vi "Invert_Binary.vi"(8 "error in (no error)":errorcluster, 11 "Input Result from Terminal":string) -> (0 "error out":errorcluster, 2 "Output Found":string[](array[string]), 3 "Result Matched?":bool)   [LabVIEW 2016]
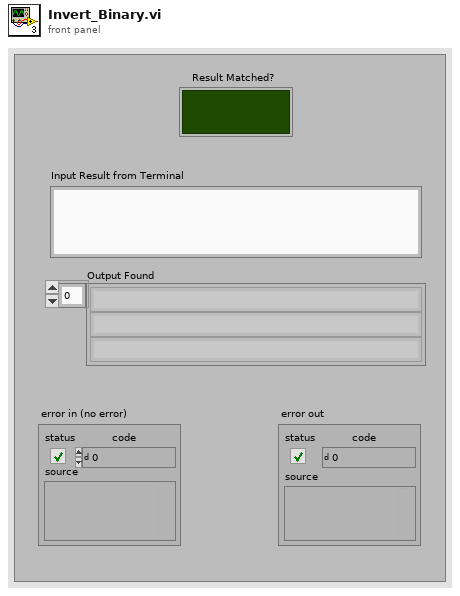
[diagram p1: front panel]
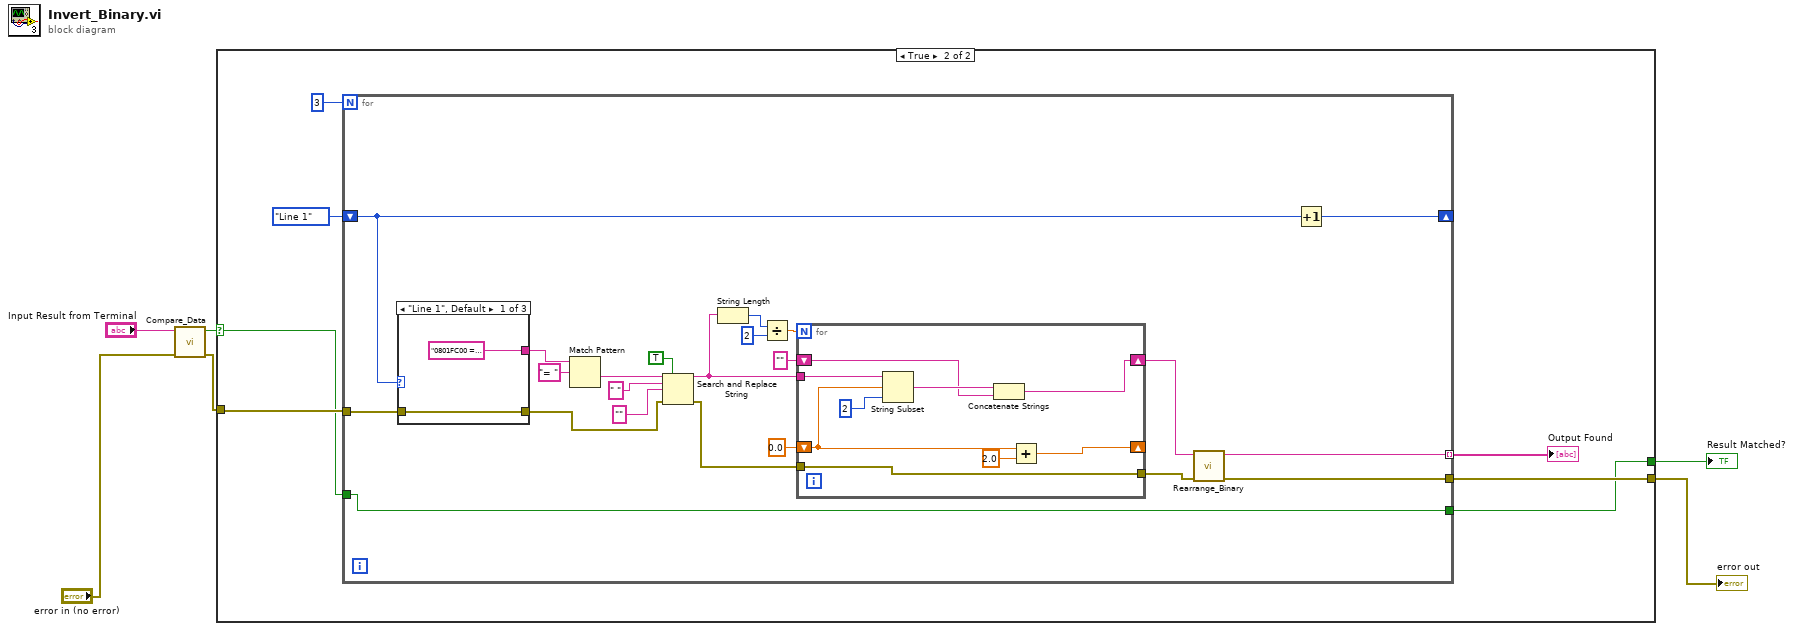
[diagram p0: block diagram]
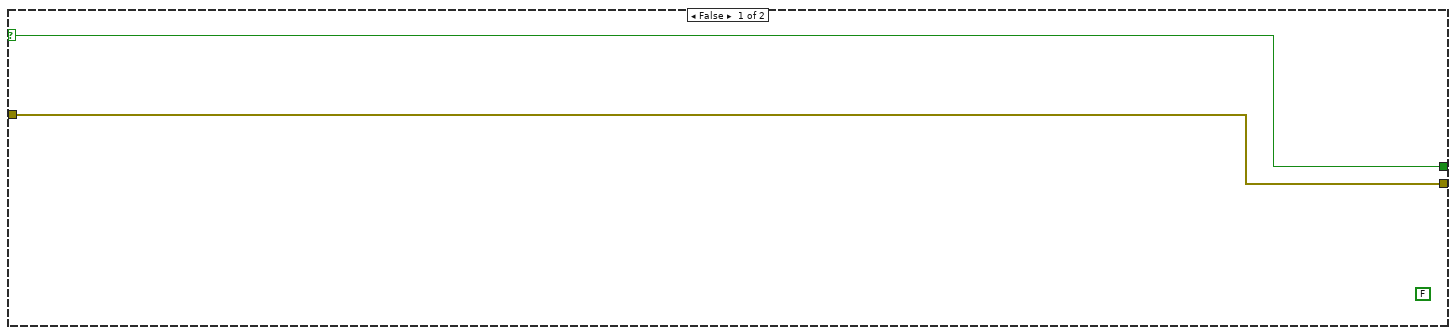
[diagram p2: hidden frame]
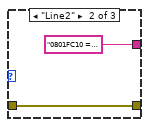
[diagram p3: hidden frame]
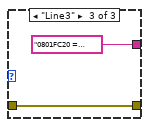
[diagram p4: hidden frame]
diagram:
  n1 = call "Compare_Data.vi"("error in (no error)"="error in (no error)", "String"="Input Result from Terminal") -> ("error out"=w3:errorcluster, "Boolean"=w5:bool)  [unwired: 8 in]
  n2 = case shown="True" w5 {
    selector: w5 -> [w8 w10]
    tunnel: w3 -> [w7 w12]
    tunnel: [w7 w11] -> w2
    tunnel: [w8 w9] -> w1
    frame False {
      (unwired) FALSE
    }
    frame True {
      n3 = for {
        N: 3 -> [_]
        shift-right: [w23] -> _
        shift-left: enum16{"Line 1", "Line2", "Line3"}."Line 1" -> [w24]
        tunnel: [w22] -> w13 mode=indexing
        tunnel: w12 -> [w21]
        tunnel: [w17] -> w11
        tunnel: w10 -> [w16]
        tunnel: [w16] -> w9
        n4 = case shown="\"Line 1\", Default" w24 {
          tunnel: ["0801FC00 = 72656D45 2D6E6F73 616C6F53 00004448" "0801FC10 = 2D4D4353 746F6F42 64616F6C 622E7265" "0801FC20 = 00006E69 00000001 00000006 00000000"] -> w37
          tunnel: w21 -> [w47 w49 w51]
          tunnel: [w47 w49 w51] -> w20
          frame "Line 1", Default {
          }
          frame "Line2" {
          }
          frame "Line3" {
          }
        }
        n5 = Match Pattern(string=w37, regular expression="= ") -> (after substring=w33:string)  [unwired: 1 in, 3 out]
        n6 = Search and Replace String(replace all?=TRUE ("replace all? (F)"), input string=w33, search string=" ", replace string="" ("replace string (\"\")"), error in=w20) -> (result string=w28:string, error out=w19:errorcluster)  [unwired: 3 in, 2 out]
        n7 = String Length(string=w28) -> (length=w29:i32)
        n8 = Divide(x=w29, y=2) -> (x/y=w34:dbl)
        n9 = for {
          N: w34 -> [_]
          shift-right: [w40] -> w26
          shift-left: "" -> [w41]
          tunnel: w28 -> [w45]
          shift-right: [w44] -> _
          shift-left: 0.0 -> [w38]
          tunnel: [w39] -> w18
          tunnel: w19 -> [w39]
          n10 = String Subset(string=w45, offset (0)=w38, length (rest)=2 ("length (rest)")) -> (substring=w42:string)
          n11 = Concatenate Strings(w42, w41) -> (w40:string)
          n12 = Add(x=w38, y=2.0) -> (x+y=w44:dbl)
        }
        n13 = call "Rearrange_Binary.vi"("error in (no error)"=w18, "String in"=w26) -> ("error out"=w17:errorcluster, "String out"=w22:string)  [unwired: 8 in]
        n14 = Increment(x=w24) -> (x+1=w23:enum16{"Line 1", "Line2", "Line3"})
      }
      "Output Found" <- w13
    }
  }
  "error out" <- w2
  "Result Matched?" <- w1
